vi "Plug_in_Cross_spectra.vi"() -> (5 "Plug in titles":string[](array[string]), 7 "Plug in values":string[](array[string]))   [LabVIEW 2013]
uses:
  Globals/Meas_global.vi
panel:
  in  "U2":u16(ring) items=["Pitot (Ur)", "XW (U)", "XW (W)", "XW  U1", "XW  U2"]
  in  "U1":u16(ring) items=["Pitot (Ur)", "XW (U)", "XW (W)", "XW  U1", "XW  U2"]
  in  "Display":bool=TRUE
  in  "Show Smoth":bool=TRUE
  in  "Save graphs":u16(ring) items=["Do not save plots", "Save plots"]
  out "U1 U2 phase":cluster{dbl, dbl, "Phase array":dbl[]}(graph)
  out "U1 U2 coherence":cluster{dbl, dbl, "Coherence array":dbl[]}(graph)
  out "U2 spectra":cluster{dbl, dbl, dbl[]}(graph)
  out "U1 spectra":cluster{dbl, dbl, dbl[]}(graph)
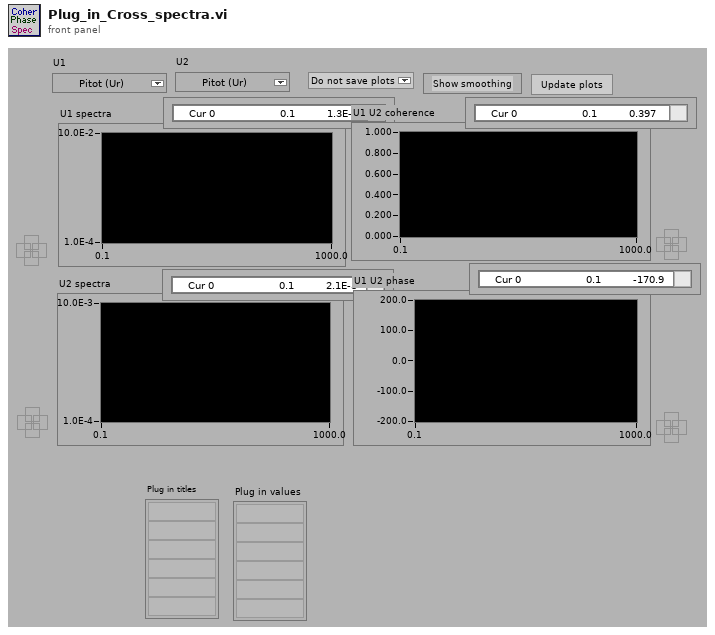
[diagram p1: front panel]
types:
  T1 = typedef "Analysis_info_cluster.ctl" = cluster{"Colour":u32, "Inst type":T2, "Inst name":string, "Symbol":string, "Code name":string, "Extra Info":string, "Inst Array":T3, "Extra Titles":string[], "Extra Values":string[], "U":dbl, "u^2":dbl, "u^3":dbl, "u^4":dbl, "Skew_u":dbl, "Kurt_u":dbl, "Sd Error in Mean":dbl, "% u'/U":dbl, "X":dbl, "Y":dbl, "Z":dbl, "Timescale integral to 25%":dbl, "Sd Error in Variance":dbl, "Calib File":path, "Calib Constants":dbl[], "Output Position":bool, "Full Stats":bool, "Av Sampling Rate":dbl, "Av No of Samples":dbl, "Total Meas Time (s)":dbl, "ADAM Ch Name":string}
  T2 = typedef "Inst_type.ctl" = enum16{"Propeller anemometer", "Raw voltage", "Pressure Transducer", "Pitot-static tube", "Preston tube", "Hot wire", "Cross wire 1", "Cross wire 2", "Generic Linear", "Generic Polynomial", "Generic BackPoly", "Fast FID", "Thermocouple", "Cold wire", "Pulsed Wire", "LDA Vel", "LDA Tran time", "LDA Arr time"}
  T3 = typedef "Instrument_Array.ctl" = enum16{"PWA", "LDA", "Analogue"}
  T4 = typedef "Time_Trace_Cluster.ctl" = cluster{"Weighting":dbl[], "Time (s)":dbl[], "Voltage":dbl[], "Eng Values":dbl[]}
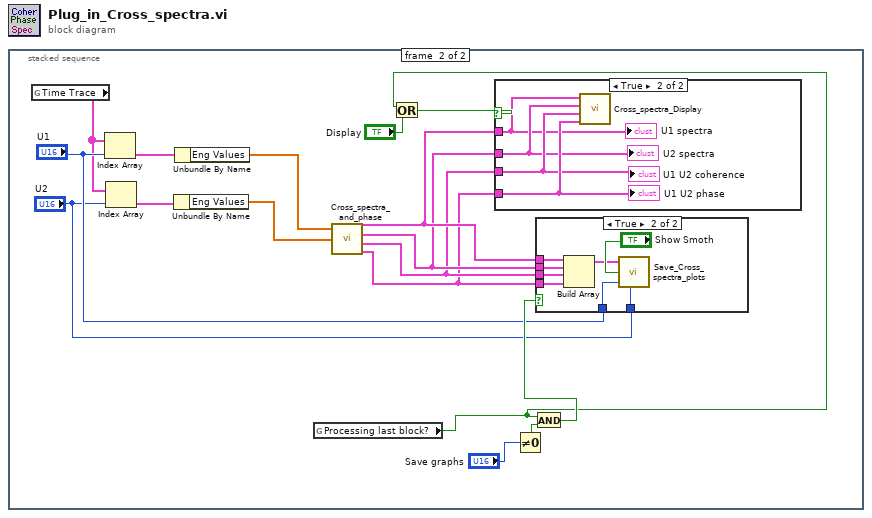
[diagram p0: block diagram]
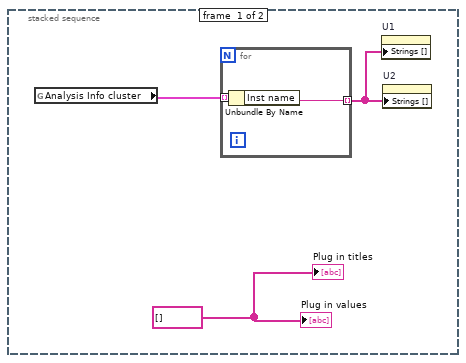
[diagram p2: hidden frame]
diagram:
  n1 = stacked-sequence {
    frame #0 {
      w1 = string[] [] ("Add in values")
      n2 = global read "Meas_global.vi" "Analysis Info cluster"() -> (w3:T1[])
      n3 = for {
        tunnel: w3 -> [w5] mode=indexing
        tunnel: [w4] -> w2 mode=indexing
        n4 = Unbundle By Name(w5) -> ("Inst name"=w4:string)
      }
      n5 = property on="U1" class="Ring (strict)"("Strings []"=w2) -> ()  [unwired: 2 in, 2 out]
      n6 = property on="U2" class="Ring (strict)"("Strings []"=w2) -> ()  [unwired: 2 in, 2 out]
      "Plug in titles" <- w1
      "Plug in values" <- w1
    }
    frame #1 {
      n7 = global read "Meas_global.vi" "Time Trace"() -> (w10:T4[])
      n8 = Index Array(array=w10, index="U1") -> (element=w9:T4)
      n9 = Index Array(array=w10, index="U2") -> (element=w7:T4)
      n10 = Unbundle By Name(w7) -> ("Eng Values"=w6:dbl[])
      n11 = Unbundle By Name(w9) -> ("Eng Values"=w8:dbl[])
      n12 = global read "Meas_global.vi" "Processing last block?"() -> (w11:bool)
      n13 = call "Cross_spectra_and_phase.vi"("U1"=w8, "U2"=w6) -> ("U1 spectra"=w15:cluster{dbl, dbl, dbl[]}, "U2 spectra"=w14:cluster{dbl, dbl, dbl[]}, "U1 U2 coherence"=w13:cluster{dbl, dbl, "Coherence array":dbl[]}, "U1 U2 phase"=w12:cluster{dbl, dbl, "Phase array":dbl[]})  [unwired: 3 out]
      n14 = Or(x=w11, y="Display") -> (x .or. y?=w19:bool)
      n15 = case shown="True" w19 {
        tunnel: w15 -> [_ w23]
        tunnel: w14 -> [_ w24]
        tunnel: w13 -> [_ w25]
        tunnel: w12 -> [_ w26]
        frame False {
        }
        frame True {
          n16 = call "Cross_spectra_Display.vi"("U1 U2 phase"=w26, "U1 U2 coherence"=w25, "U2 spectra"=w24, "U1 spectra"=w23) -> ()  [unwired: 4 out]
          "U1 spectra" <- w23
          "U2 spectra" <- w24
          "U1 U2 coherence" <- w25
          "U1 U2 phase" <- w26
        }
      }
      n17 = Not Equal To 0?(x="Save graphs") -> (x != 0?=w21:bool)
      n18 = And(x=w11, y=w21) -> (x .and. y?=w20:bool)
      n19 = case shown="True" w20 {
        tunnel: "U1" -> [_ w33]
        tunnel: "U2" -> [_ w32]
        tunnel: w15 -> [_ w30]
        tunnel: w14 -> [_ w29]
        tunnel: w13 -> [_ w28]
        tunnel: w12 -> [_ w27]
        frame False {
        }
        frame True {
          n20 = Build Array(w30, w29, w28, w27) -> (w31:cluster{dbl, dbl, "Phase array":dbl[]}[])
          n21 = call "Save_Cross_spectra_plots.vi"("Plots to save"=w31, "Show Smooth"="Show Smoth", "U1"=w33, "U2"=w32) -> ()  [unwired: 1 in, 2 out]
        }
      }
    }
  }
